vi "Check Network Connection.vi"(9 "CD Path":string, 10 "IP Address":string, 11 "Comm Ref":T1) -> (0 "error out":errorcluster, 3 "Comm Ref":T1)   [LabVIEW 2013, in "PID Control Workspace Tool.lvlib"]
uses:
  PID Control Workspace Tool.lvlib
  <vilib>/NI Veristand/Execution/CustomDevice/Custom Device Ref.ctl
  NationalInstruments.VeriStand.ClientAPI
  <vilib>/NI VeriStand/Execution/CustomDevice/NI_VS Custom Device ExecutionAPI.lvlib
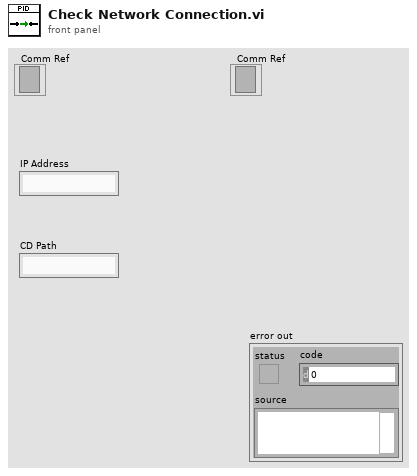
[diagram p1: front panel]
types:
  T1 = typedef "NI_VS Custom Device ExecutionAPI.lvlib/Custom Device Ref.ctl" = refnum<k24>
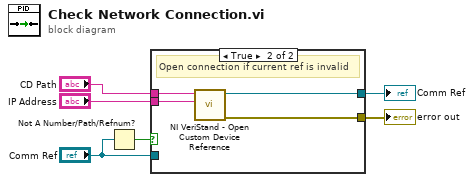
[diagram p0: block diagram]
diagram:
  n1 = Not A Number/Path/Refnum?(number/path/refnum="Comm Ref") -> (NaN/Path/Refnum?=w5:bool)
  n2 = case shown="True" w5 {
    tunnel: "Comm Ref" -> [w7 _]
    tunnel: [_ w9] -> w6
    tunnel: "IP Address" -> [_ w11]
    tunnel: "CD Path" -> [_ w10]
    tunnel: [w7 w8] -> w2
    frame False {
      # "Current connection ref valid"
    }
    frame True {
      # "Open connection if current ref is invalid"
      n3 = call <vilib>:"NI VeriStand - Open Custom Device Reference.vi"("Gateway IP Address (\"\": localhost)"=w11, "Custom Device Path"=w10) -> ("error out"=w9:errorcluster, "Custom Device"=w8:T1)  [unwired: 8 in]
    }
  }
  "error out" <- w6
  "Comm Ref" <- w2
